vi "CspecH2O_2024.vi"(0 "Temperature [K]":dbl=293.4405 format="%.4g") -> (1 "rel. unc. Cp0/R water":dbl=0.001 format="%.2e", 2 "Cp0/R water":dbl=4.037217363253289, 3 "Cp0 [J / Kmol]":dbl=33.567292774840084, 4 "Cv0 [J / Kmol]":dbl=25.252830174840085, 5 "Gamma0 water":dbl=1.329248743306557)   [LabVIEW 2016]
panel:
  out "abs unc Cp0/R water":dbl=0.0020186086816266443 format="%#.4g"
  in  "rel. unc. Cp0/R water":dbl=0.001 format="%.2e"
  # "from IAPWS95 [19] Eq. 5.6 with coeffs in Table 6.1, based on spectroscopic data by Woolley and calcs. by Cooper - uncertainty estimate at 0.1% level by comparison of the relative difference between the eqaution and various data sources (Woolley diff. years, Gurvich) between 200 K and 600 K as in Fig. 4.7 of [19]. \nThe value reported by Zuckerwar at 300.00 K using Touloukian interpolation is relatively different by 0.03 %. This value is coincident with Touloukian interpolation of 1970, with the coefficients reported by Zuckerwar (Table 3.1 vol. I)"
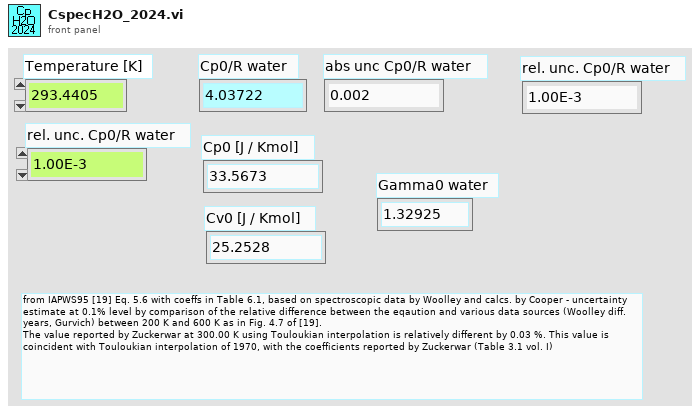
[diagram p1: front panel]
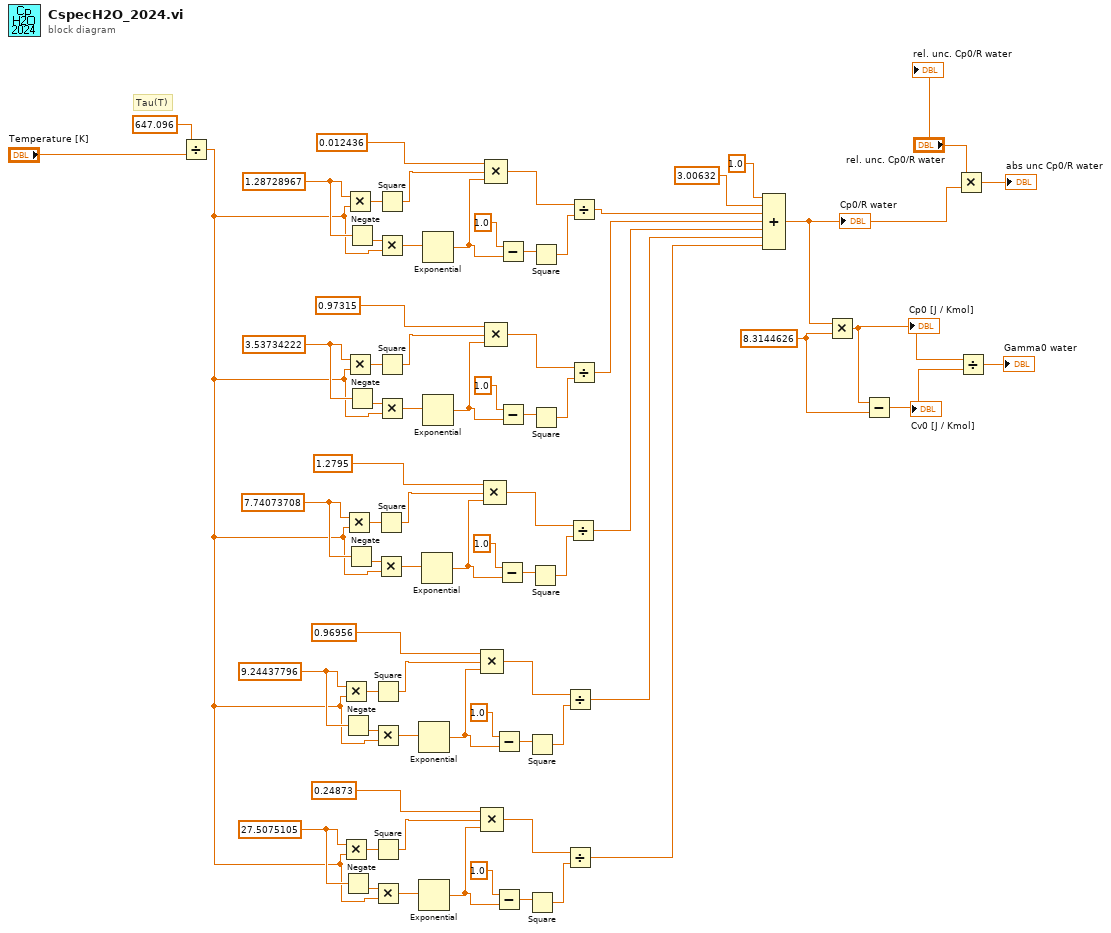
[diagram p0: block diagram]
diagram:
  w7 = 8.3144626
  w21 = 27.5075105
  w32 = 9.24437796
  w43 = 7.74073708
  w54 = 3.53734222
  w65 = 1.28728967
  # "Tau(T)"
  n1 = Divide(x=647.096, y="Temperature [K]") -> (x/y=w13:dbl)
  n2 = Multiply(x=w32, y=w13) -> (x*y=w34:dbl)
  n3 = Multiply(x=w21, y=w13) -> (x*y=w23:dbl)
  n4 = Negate(x=w32) -> (-x=w31:dbl)
  n5 = Negate(x=w21) -> (-x=w20:dbl)
  n6 = Multiply(x=w43, y=w13) -> (x*y=w45:dbl)
  n7 = Multiply(x=w65, y=w13) -> (x*y=w67:dbl)
  n8 = Multiply(x=w54, y=w13) -> (x*y=w56:dbl)
  n9 = Negate(x=w43) -> (-x=w42:dbl)
  n10 = Negate(x=w65) -> (-x=w64:dbl)
  n11 = Negate(x=w54) -> (-x=w53:dbl)
  n12 = Square(x=w34) -> (x^2=w33:dbl)
  n13 = Multiply(x=w31, y=w13) -> (x*y=w30:dbl)
  n14 = Square(x=w23) -> (x^2=w22:dbl)
  n15 = Multiply(x=w20, y=w13) -> (x*y=w19:dbl)
  n16 = Square(x=w45) -> (x^2=w44:dbl)
  n17 = Multiply(x=w42, y=w13) -> (x*y=w41:dbl)
  n18 = Square(x=w67) -> (x^2=w66:dbl)
  n19 = Multiply(x=w64, y=w13) -> (x*y=w63:dbl)
  n20 = Square(x=w56) -> (x^2=w55:dbl)
  n21 = Multiply(x=w53, y=w13) -> (x*y=w52:dbl)
  n22 = Exponential(1:w30) -> (0:w27:dbl)
  n23 = Exponential(1:w19) -> (0:w16:dbl)
  n24 = Exponential(1:w41) -> (0:w38:dbl)
  n25 = Exponential(1:w63) -> (0:w60:dbl)
  n26 = Exponential(1:w52) -> (0:w49:dbl)
  n27 = Compound Arithmetic op=MULTIPLY(0.96956, w33, w27) -> (w29:dbl)
  n28 = Compound Arithmetic op=MULTIPLY(0.24873, w22, w16) -> (w18:dbl)
  n29 = Compound Arithmetic op=MULTIPLY(1.2795, w44, w38) -> (w40:dbl)
  n30 = Compound Arithmetic op=MULTIPLY(0.012436, w66, w60) -> (w62:dbl)
  n31 = Compound Arithmetic op=MULTIPLY(0.97315, w55, w49) -> (w51:dbl)
  n32 = Subtract(x=1.0, y=w27) -> (x-y=w26:dbl)
  n33 = Subtract(x=1.0, y=w16) -> (x-y=w15:dbl)
  n34 = Subtract(x=1.0, y=w38) -> (x-y=w37:dbl)
  n35 = Subtract(x=1.0, y=w60) -> (x-y=w59:dbl)
  n36 = Subtract(x=1.0, y=w49) -> (x-y=w48:dbl)
  n37 = Square(x=w26) -> (x^2=w25:dbl)
  n38 = Square(x=w15) -> (x^2=w14:dbl)
  n39 = Square(x=w37) -> (x^2=w36:dbl)
  n40 = Square(x=w59) -> (x^2=w58:dbl)
  n41 = Square(x=w48) -> (x^2=w47:dbl)
  n42 = Divide(x=w29, y=w25) -> (x/y=w9:dbl)
  n43 = Divide(x=w18, y=w14) -> (x/y=w8:dbl)
  n44 = Divide(x=w40, y=w36) -> (x/y=w10:dbl)
  n45 = Divide(x=w62, y=w58) -> (x/y=w12:dbl)
  n46 = Divide(x=w51, y=w47) -> (x/y=w11:dbl)
  n47 = Compound Arithmetic op=ADD(1.0 ("value"), 3.00632, w12, w11, w10, w9, w8) -> (w2:dbl)
  "Cp0/R water" <- w2
  n48 = Multiply(x=w2, y=w7) -> (x*y=w6:dbl)
  "Cp0 [J / Kmol]" <- w6
  n49 = Subtract(x=w6, y=w7) -> (x-y=w5:dbl)
  "Cv0 [J / Kmol]" <- w5
  n50 = Multiply(x="rel. unc. Cp0/R water", y=w2) -> (x*y=→"abs unc Cp0/R water":dbl)
  n51 = Divide(x=w6, y=w5) -> (x/y=→"Gamma0 water":dbl)
  "rel. unc. Cp0/R water" <- "rel. unc. Cp0/R water"
